vi "VCC_controle_rpm_compressor.vi"() -> ()   [LabVIEW 2019]
uses:
  <vilib>/DAQmx/write.llb/DAQmx Write (Counter Frequency 1Chan 1Samp).vi
  <vilib>/DAQmx/configure/timing.llb/DAQmx Timing (Implicit).vi
  <vilib>/DAQmx/miscellaneous.llb/DAQmx Fill In Error Info.vi
panel:
  in  "task/channels in":refnum<k21>="VCC"
  out "Tempo While VCC":u32=1000
  in  "RPM":i32=3600
  in  "Stop":bool
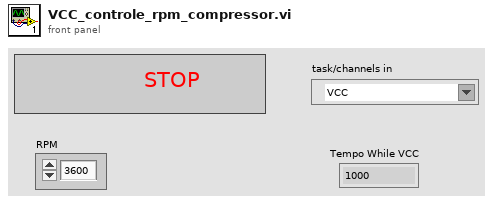
[diagram p1: front panel]
diagram:
  w1 = 10123 items=["Finite Samples"=10178, "Continuous Samples"=10123, "Hardware Timed Single Point"=12522] ("sample mode")
  n1 = call-poly <vilib>:"DAQmx Timing.vi"("task/channels in"="task/channels in", "sample mode"=w1) -> ("task out"=w3:refnum<k21>, "error out"=w2:errorcluster)  [unwired: 12 in]
  n2 = call <vilib>:"DAQmx Start Task.vi"("task/channels in"=w3, "error in"=w2) -> ("task out"=w10:refnum<k21>, "error out"=w9:errorcluster)  [unwired: 12 in]
  n3 = while {
    tunnel: w10 -> [w30]
    tunnel: [w29] -> w8
    tunnel: [w28] -> w7
    tunnel: w9 -> [w27]
    stop <- w12 stop-if-true
    # "VCC"
    n4 = local read "Stop"() -> (w12:bool)
    n5 = In Range and Coerce(upper limit=4500, x="RPM", lower limit=1600) -> (coerced(x)=w18:i32, In Range?=w14:bool)
    n6 = Not(x=w14) -> (.not. x?=w13:bool)
    n7 = Or(x=w13, y=w12) -> (x .or. y?=w11:bool)
    n8 = Wait (ms)(milliseconds to wait=u32 1000) -> ()  [unwired: 1 out]
    n9 = case shown="True" w11 {
      tunnel: w18 -> [w31 _]
      tunnel: [w31 1 ("upper limit")] -> w16
      frame False {
      }
      frame True {
      }
    }
    n10 = feedback #1() -> (w23:u32)  [unwired: 1 in]
    n11 = Tick Count (ms)() -> (millisecond timer value=w22:u32)
    n12 = feedback-in #1(w22) -> ()
    n13 = Subtract(x=w22, y=w23) -> (x-y=→"Tempo While VCC":u32)
    n14 = Divide(x=w16, y=30.0) -> (x/y=w15:dbl)
    n15 = call-poly <vilib>:"DAQmx Write.vi"("task/channels in"=w30, "frequency"=w15, "duty cycle"=0.5, "error in"=w27) -> ("task out"=w29:refnum<k21>, "error out"=w28:errorcluster)  [unwired: 9 in, 1 out]
  }
  n16 = call <vilib>:"DAQmx Stop Task.vi"("task/channels in"=w8, "error in"=w7) -> ("task out"=w6:refnum<k21>, "error out"=w5:errorcluster)  [unwired: 12 in]
  n17 = call <vilib>:"DAQmx Clear Task.vi"("task in"=w6, "error in"=w5) -> ()  [unwired: 13 in, 1 out]
